vi "TCS_CFN_VS50BR_v2.vi"() -> ()   [LabVIEW 2011]
uses:
  <vilib>/Instr/_visa.llb/VISA Configure Serial Port (Instr).vi
panel:
  in  "LP_X-Up 4":sgl(slide) scale=-180.0..180.0
  in  "LP_Y-Easth 4":sgl(slide)=0.128098 scale=-180.0..180.0
  in  "LP_Z-North 4":sgl(slide)=0.467339 scale=-180.0..180.0
  in  "Height 4":sgl(slide)=622.367 scale=-2000.0..10000.0
  in  "Longitude 4":sgl(slide)=-45.860622 scale=-180.0..180.0
  in  "Latitude  2":sgl(slide)=-23.213156 scale=-90.0..90.0
  in  "Azimuth 4":sgl(slide) scale=0.0..360.0
  in  "Offset Pitch 4":sgl(slide) scale=-180.0..180.0
  in  "Offset Roll 4":sgl(slide) scale=-180.0..180.0
  in  "Offset Yaw 4":sgl(slide) scale=-180.0..180.0
  in  "Send":bool
  in  "LP_X-Up 3":sgl(slide) scale=-180.0..180.0
  in  "LP_Y-Easth 3":sgl(slide)=0.128098 scale=-180.0..180.0
  in  "LP_Z-North 3":sgl(slide)=0.467339 scale=-180.0..180.0
  in  "Height 3":sgl(slide)=622.367 scale=-2000.0..10000.0
  in  "Longitude 3":sgl(slide)=-45.860622 scale=-180.0..180.0
  in  "Latitude  2":sgl(slide)=-23.213156 scale=-90.0..90.0
  in  "Azimuth 3":sgl(slide) scale=0.0..360.0
  in  "Offset Pitch 3":sgl(slide) scale=-180.0..180.0
  in  "Offset Roll 3":sgl(slide) scale=-180.0..180.0
  in  "Offset Yaw 3":sgl(slide) scale=-180.0..180.0
  in  "Init":bool
  in  "LP_X-Up 2":sgl(slide) scale=-180.0..180.0
  in  "LP_Y-Easth 2":sgl(slide)=0.128098 scale=-180.0..180.0
  in  "LP_Z-North 2":sgl(slide)=0.467339 scale=-180.0..180.0
  in  "Height 2":sgl(slide)=622.367 scale=-2000.0..10000.0
  in  "Longitude 2":sgl(slide)=-45.860622 scale=-180.0..180.0
  in  "Latitude  2":sgl(slide)=-23.213156 scale=-90.0..90.0
  in  "Azimuth 2":sgl(slide) scale=0.0..360.0
  in  "Offset Pitch 2":sgl(slide) scale=-180.0..180.0
  in  "Offset Roll 2":sgl(slide) scale=-180.0..180.0
  in  "Offset Yaw 2":sgl(slide) scale=-180.0..180.0
  in  "Tab Control 4":enum32{"TCS_Utility", "TCS_Utility 2"}(tab)
  in  "Fact Reserved":bool
  in  "Download":bool
  in  "Fact Config":bool
  in  "NavOn":bool
  out "Half Second":bool[][](array[boolean])=[[FALSE, FALSE, FALSE, FALSE, FALSE, FALSE, FALSE, FALSE, FALSE, FALSE], [FALSE, FALSE, TRUE, TRUE, TRUE, TRUE, TRUE, FALSE, FALSE, FALSE], [FALSE, TRUE, FALSE, FALSE, FALSE, FALSE, FALSE, TRUE, FALSE, FALSE], [FALSE, TRUE, FALSE, FALSE, FALSE, FALSE, FALSE, TRUE, FALSE, FALSE], [FALSE, TRUE, FALSE, FALSE, FALSE, FALSE, FALSE, TRUE, FALSE, FALSE], [FALSE, TRUE, FALSE, FALSE, FALSE, FALSE, FALSE, TRUE, FALSE, FALSE], [FALSE, TRUE, FALSE, FALSE, FALSE, FALSE, FALSE, TRUE, FALSE, FALSE], [FALSE, TRUE, FALSE, FALSE, FALSE, FALSE, FALSE, TRUE, FALSE, FALSE], [FALSE, FALSE, TRUE, TRUE, TRUE, TRUE, TRUE, FALSE, FALSE, FALSE], [FALSE, FALSE, FALSE, FALSE, FALSE, FALSE, FALSE, FALSE, FALSE, FALSE]]
  out "Min 1":bool[][](array[boolean])=[[FALSE, FALSE, FALSE, FALSE, FALSE, FALSE, FALSE, FALSE, FALSE, FALSE], [FALSE, FALSE, TRUE, TRUE, TRUE, TRUE, TRUE, FALSE, FALSE, FALSE], [FALSE, TRUE, FALSE, FALSE, FALSE, FALSE, FALSE, TRUE, FALSE, FALSE], [FALSE, TRUE, FALSE, FALSE, FALSE, FALSE, FALSE, TRUE, FALSE, FALSE], [FALSE, TRUE, FALSE, FALSE, FALSE, FALSE, FALSE, TRUE, FALSE, FALSE], [FALSE, TRUE, FALSE, FALSE, FALSE, FALSE, FALSE, TRUE, FALSE, FALSE], [FALSE, TRUE, FALSE, FALSE, FALSE, FALSE, FALSE, TRUE, FALSE, FALSE], [FALSE, TRUE, FALSE, FALSE, FALSE, FALSE, FALSE, TRUE, FALSE, FALSE], [FALSE, FALSE, TRUE, TRUE, TRUE, TRUE, TRUE, FALSE, FALSE, FALSE], [FALSE, FALSE, FALSE, FALSE, FALSE, FALSE, FALSE, FALSE, FALSE, FALSE]]
  out "Min 0":bool[][](array[boolean])=[[FALSE, FALSE, FALSE, FALSE, FALSE, FALSE, FALSE, FALSE, FALSE, FALSE], [FALSE, FALSE, TRUE, TRUE, TRUE, TRUE, TRUE, FALSE, FALSE, FALSE], [FALSE, TRUE, FALSE, FALSE, FALSE, FALSE, FALSE, TRUE, FALSE, FALSE], [FALSE, TRUE, FALSE, FALSE, FALSE, FALSE, FALSE, TRUE, FALSE, FALSE], [FALSE, TRUE, FALSE, FALSE, FALSE, FALSE, FALSE, TRUE, FALSE, FALSE], [FALSE, TRUE, FALSE, FALSE, FALSE, FALSE, FALSE, TRUE, FALSE, FALSE], [FALSE, TRUE, FALSE, FALSE, FALSE, FALSE, FALSE, TRUE, FALSE, FALSE], [FALSE, TRUE, FALSE, FALSE, FALSE, FALSE, FALSE, TRUE, FALSE, FALSE], [FALSE, FALSE, TRUE, TRUE, TRUE, TRUE, TRUE, FALSE, FALSE, FALSE], [FALSE, FALSE, FALSE, FALSE, FALSE, FALSE, FALSE, FALSE, FALSE, FALSE]]
  out "Hour 1":bool[][](array[boolean])=[[FALSE, FALSE, FALSE, FALSE, FALSE, FALSE, FALSE, FALSE, FALSE, FALSE], [FALSE, FALSE, TRUE, TRUE, TRUE, TRUE, TRUE, FALSE, FALSE, FALSE], [FALSE, TRUE, FALSE, FALSE, FALSE, FALSE, FALSE, TRUE, FALSE, FALSE], [FALSE, TRUE, FALSE, FALSE, FALSE, FALSE, FALSE, TRUE, FALSE, FALSE], [FALSE, TRUE, FALSE, FALSE, FALSE, FALSE, FALSE, TRUE, FALSE, FALSE], [FALSE, TRUE, FALSE, FALSE, FALSE, FALSE, FALSE, TRUE, FALSE, FALSE], [FALSE, TRUE, FALSE, FALSE, FALSE, FALSE, FALSE, TRUE, FALSE, FALSE], [FALSE, TRUE, FALSE, FALSE, FALSE, FALSE, FALSE, TRUE, FALSE, FALSE], [FALSE, FALSE, TRUE, TRUE, TRUE, TRUE, TRUE, FALSE, FALSE, FALSE], [FALSE, FALSE, FALSE, FALSE, FALSE, FALSE, FALSE, FALSE, FALSE, FALSE]]
  out "Hour 0":bool[][](array[boolean])=[[FALSE, FALSE, FALSE, FALSE, FALSE, FALSE, FALSE, FALSE, FALSE, FALSE], [FALSE, FALSE, TRUE, TRUE, TRUE, TRUE, TRUE, FALSE, FALSE, FALSE], [FALSE, TRUE, FALSE, FALSE, FALSE, FALSE, FALSE, TRUE, FALSE, FALSE], [FALSE, TRUE, FALSE, FALSE, FALSE, FALSE, FALSE, TRUE, FALSE, FALSE], [FALSE, TRUE, FALSE, FALSE, FALSE, FALSE, FALSE, TRUE, FALSE, FALSE], [FALSE, TRUE, FALSE, FALSE, FALSE, FALSE, FALSE, TRUE, FALSE, FALSE], [FALSE, TRUE, FALSE, FALSE, FALSE, FALSE, FALSE, TRUE, FALSE, FALSE], [FALSE, TRUE, FALSE, FALSE, FALSE, FALSE, FALSE, TRUE, FALSE, FALSE], [FALSE, FALSE, TRUE, TRUE, TRUE, TRUE, TRUE, FALSE, FALSE, FALSE], [FALSE, FALSE, FALSE, FALSE, FALSE, FALSE, FALSE, FALSE, FALSE, FALSE]]
  in  "Stop":bool
  out "string in":string
  out "string out":string
  out "DV_Word":bool[](array[boolean])
  out "B_55":u8 format="%x"
  out "B_54":u8 format="%x"
  out "String":string
  in  "Tab Control":enum32{"Page 1", "Page 2", "Page 3"}(tab)
  in  "Offset Yaw":sgl(slide) scale=-180.0..180.0
  in  "Offset Roll":sgl(slide) scale=-180.0..180.0
  in  "Offset Pitch":sgl(slide) scale=-180.0..180.0
  in  "Longitude":sgl(slide)=-45.860622 scale=-180.0..180.0
  in  "Latitude":sgl(slide)=-23.213156 scale=-90.0..90.0
  in  "Azimuth":sgl(slide) scale=0.0..360.0
  in  "Height":sgl(slide)=622.367 scale=-2000.0..10000.0
  in  "LP_X-Up":sgl(slide) scale=-180.0..180.0
  in  "LP_Y-Easth":sgl(slide)=0.128098 scale=-180.0..180.0
  in  "LP_Z-North":sgl(slide)=0.467339 scale=-180.0..180.0
  # "B#55 (Configuration and Command Mode)"
  # "0x35"
  # "0xBD"
  # "0XFA"
  # "0XEE"
  # "0XAB"
  # "B#54 (Data Validity Word)"
  # "1= Installation Offset input valid data\n1= Launch Azimuth geodetic orientation, position, (lat, long, height) valid \n1= Velocity input valid data \nRFU\nRFU\nRFU\n 7,6     00= \"Init Cmd\" (Configuration parameters setting)\n           10= \"NAV_On\"\n           01= Reserved\n           11= Enter Configuration Mode"
  # "0\n1\n2\n3\n4\n5\n6\n7"
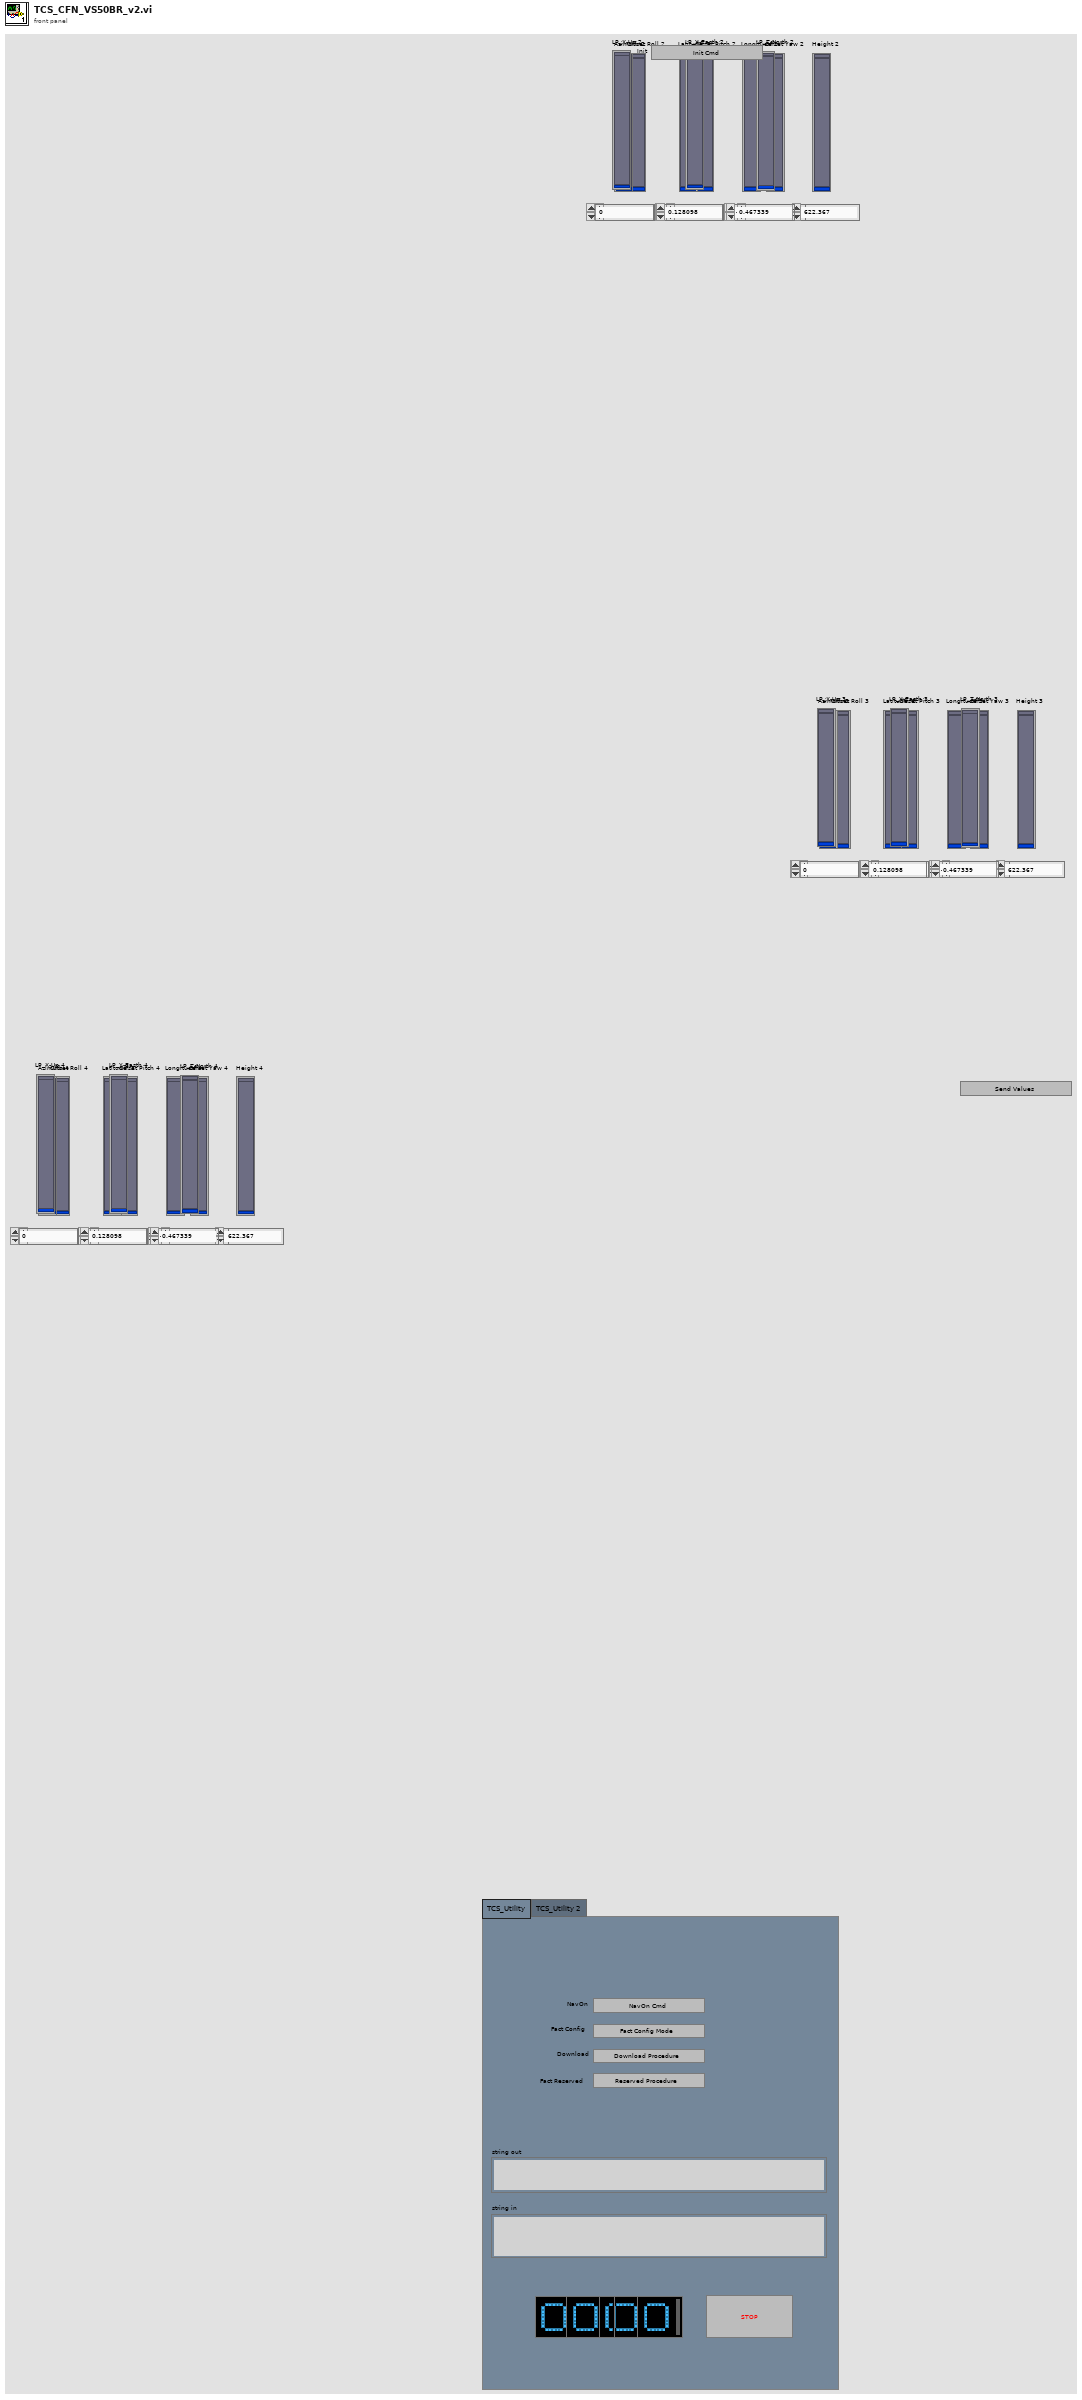
[diagram p1: front panel]
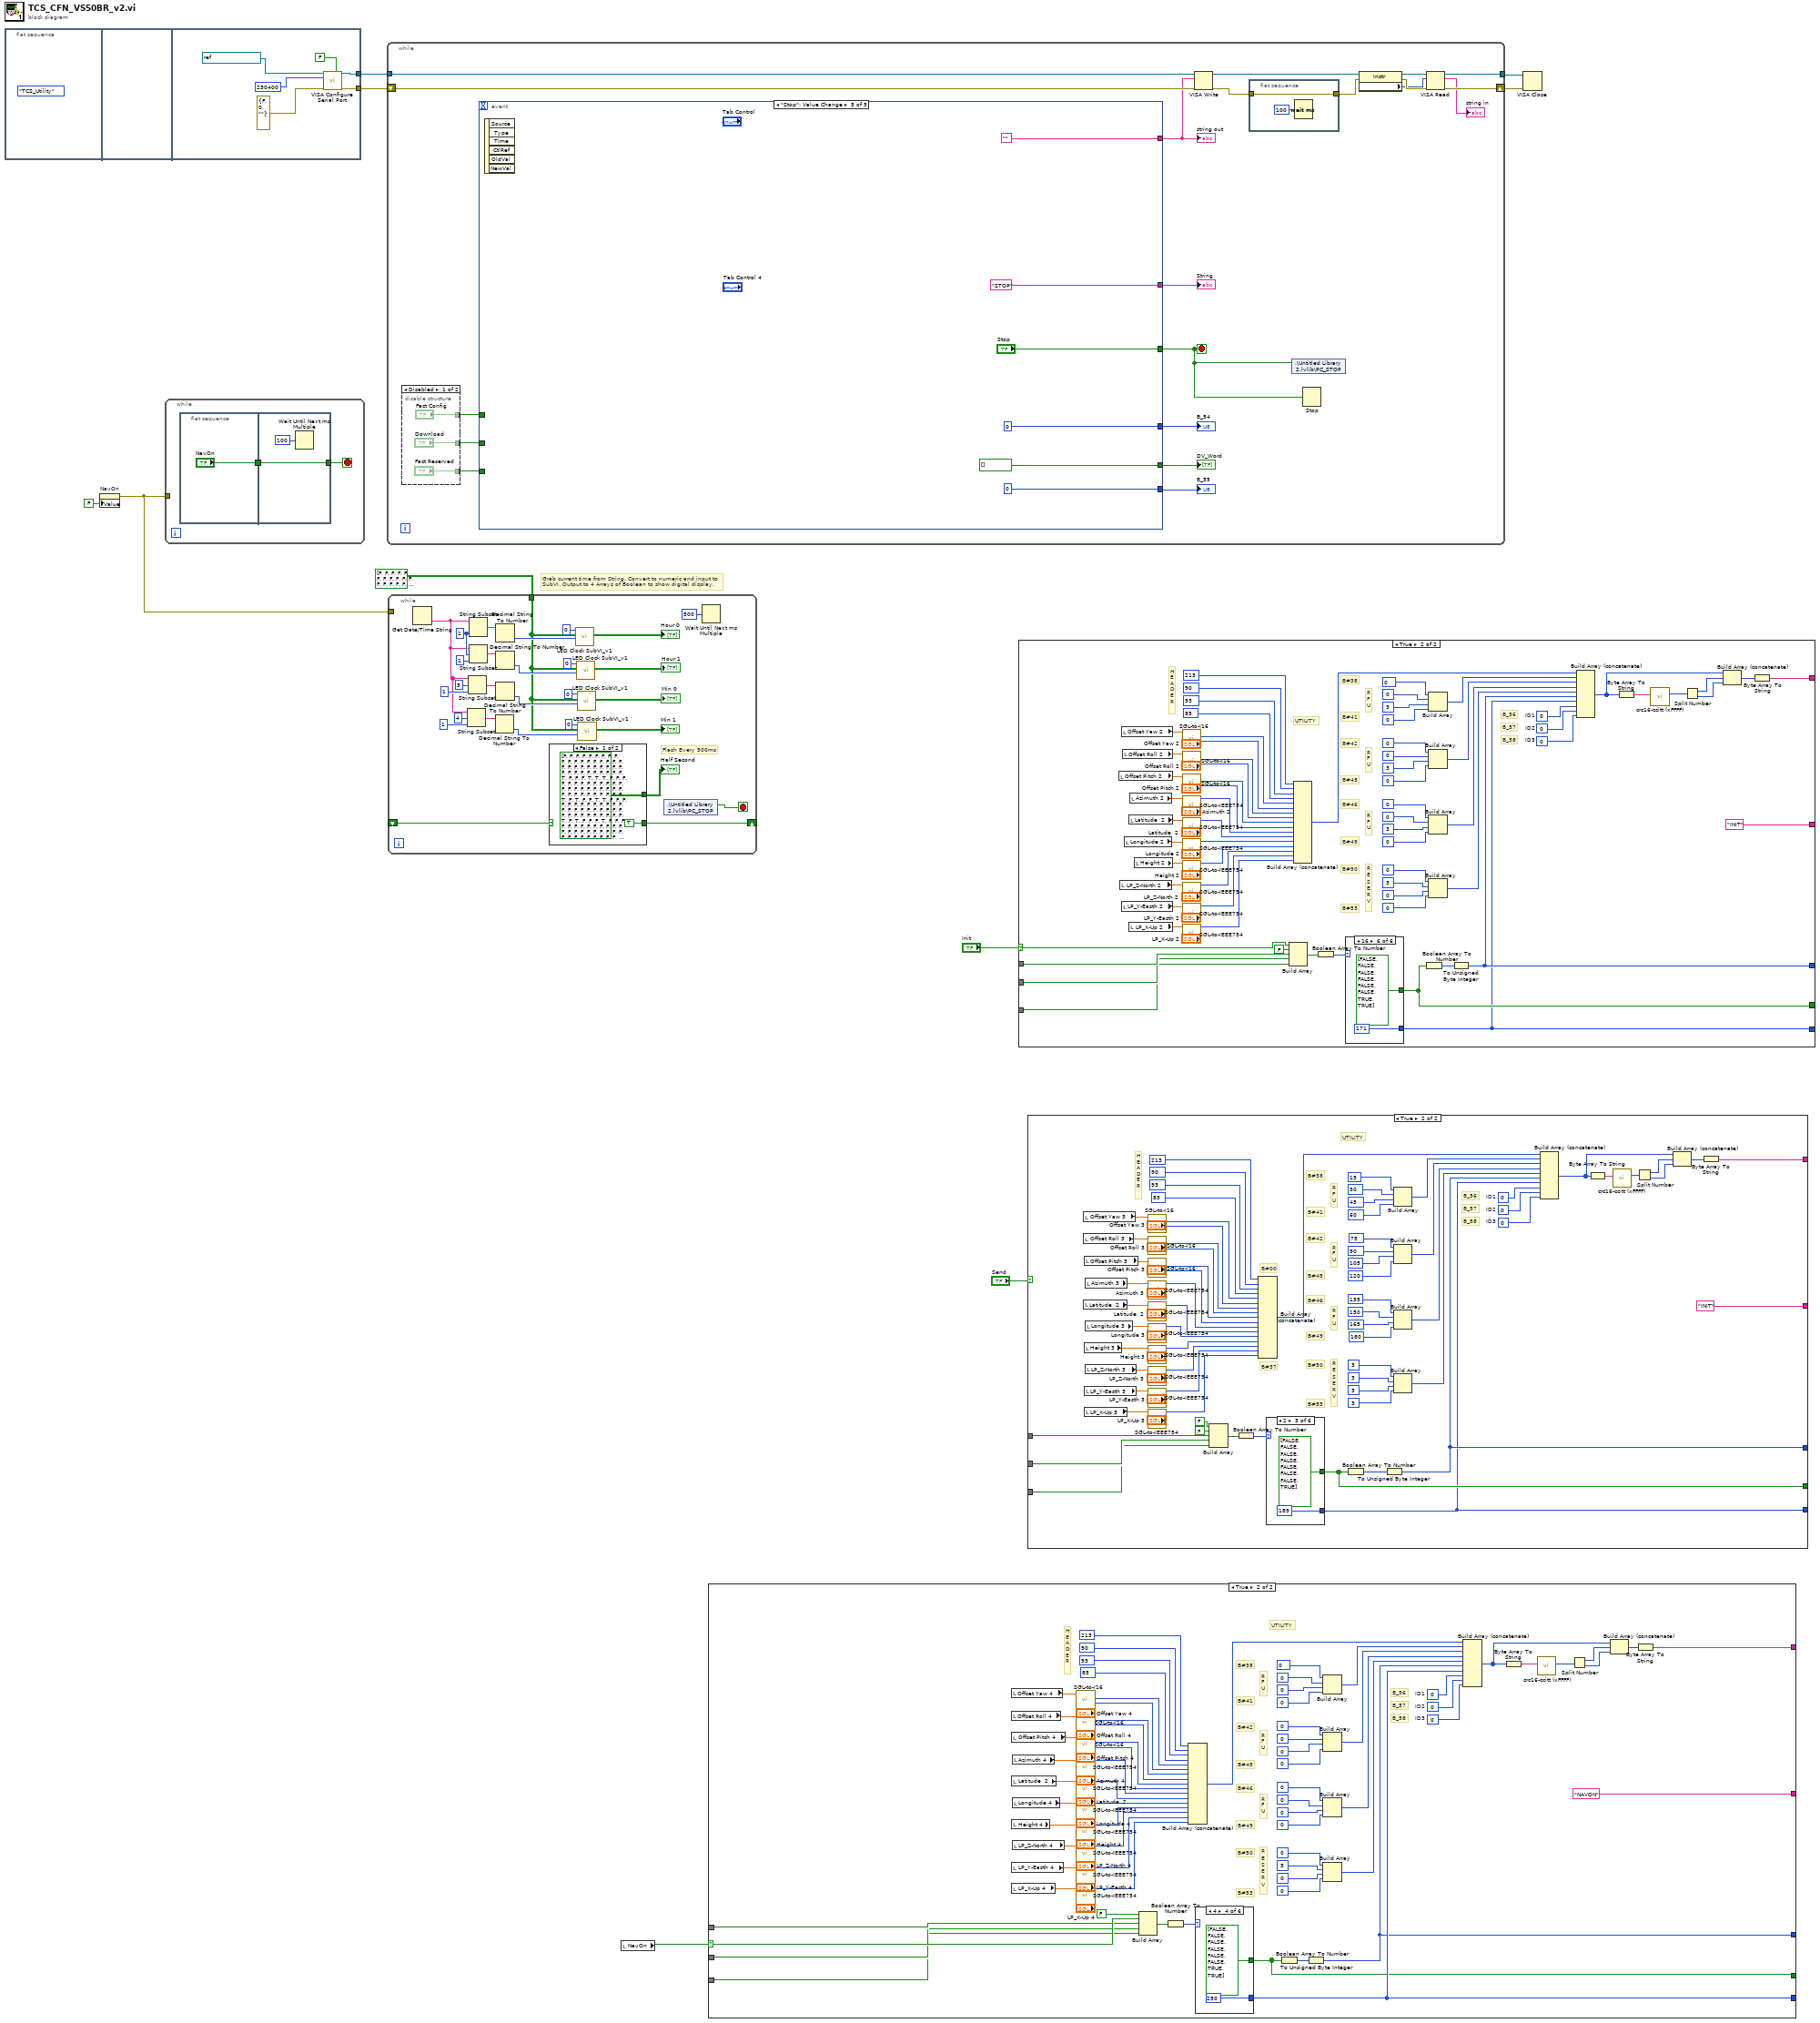
[diagram p0: block diagram]
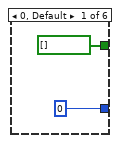
[diagram p3: hidden frame]
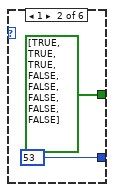
[diagram p4: hidden frame]
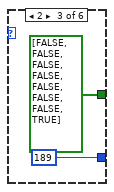
[diagram p5: hidden frame]
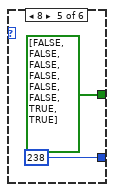
[diagram p6: hidden frame]
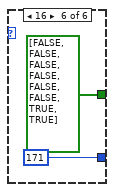
[diagram p7: hidden frame]
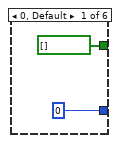
[diagram p9: hidden frame]
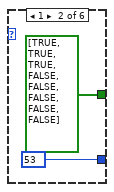
[diagram p10: hidden frame]
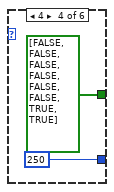
[diagram p11: hidden frame]
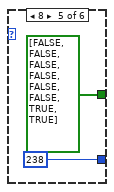
[diagram p12: hidden frame]
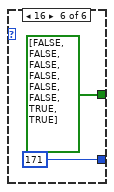
[diagram p13: hidden frame]
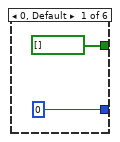
[diagram p15: hidden frame]
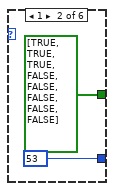
[diagram p16: hidden frame]
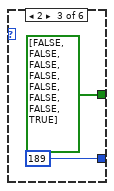
[diagram p17: hidden frame]
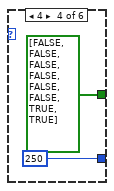
[diagram p18: hidden frame]
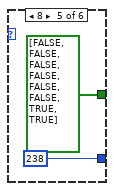
[diagram p19: hidden frame]
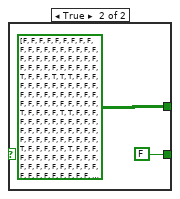
[diagram p20: hidden frame]
diagram:
  # "Grab current time from String, Convert to numeric and input to\nSubVI. Output to 4 Arrays of Boolean to show digital display."
  n1 = flat-sequence {
    tunnel: [w13] -> w10
    tunnel: [w12] -> w9
    frame #0 {
      (unwired) enum32{"TCS_Utility", "Parser"}."TCS_Utility" ("Tab Control 3")
    }
    frame #1 {
    }
    frame #2 {
      n2 = call-poly "VISA Configure Serial Port"("VISA resource name"=refnum<visa-resource-name> "ASRL3::INSTR", "Enable Termination\nChar (T)"=FALSE ("Enable Termination\nChar (T)"), "baud rate (9600)"=u32 230400 ("Serial Settings:Baud Rate"), "error in (no error)"=errorcluster {"status"=FALSE, "code"=0, "source"=""}) -> ("VISA resource name out"=w13:refnum<visa-resource-name>, "error out"=w12:errorcluster)  [unwired: 10 in]
    }
  }
  n3 = property on="NavOn" class="Bool (strict)"("Value"=FALSE ("NavOn")) -> (error out=w4:errorcluster)  [unwired: 2 in, 1 out]
  n4 = while {
    tunnel: w4 -> [_]
    stop <- w18 stop-if-true
    n5 = flat-sequence {
      tunnel: ["NavOn"] -> w17
      tunnel: [w20] -> w18
      tunnel: w17 -> [w20]
      frame #0 {
      }
      frame #1 {
        n6 = Wait Until Next ms Multiple(millisecond multiple=u32 100) -> ()  [unwired: 1 out]
      }
    }
  }
  n7 = while {
    tunnel: w10 -> [w34]
    tunnel: [w24] -> w8
    shift-right: [w25] -> w7
    shift-left: w9 -> [w33]
    stop <- w22 stop-if-true
    n8 = disable-structure shown="Disabled" {
      disable-tunnel: ["Fact Config" _] -> w41
      disable-tunnel: ["Download" _] -> w40
      disable-tunnel: ["Fact Reserved" _] -> w39
      frame Disabled {
      }
      frame Enabled {
      }
    }
    n9 = event shown="[4] \"Stop\": Value Change" {
      selector: _ -> [_ _ _ _ _]
      dyn-events: _ -> [_ _ _ _ _]
      timeout: _ -> [_ _ _ _ _]
      tunnel: ["" _ w50 w51 ""] -> w32
      tunnel: w41 -> [_ _ _ _ _]
      tunnel: w40 -> [_ _ _ _ _]
      tunnel: w39 -> [_ _ _ _ _]
      tunnel: [u8 0 _ _ _ u8 0] -> w38
      tunnel: [bool[] [] ("DV_Word") _ _ _ bool[] [] ("DV_Word")] -> w37
      tunnel: [u8 0 _ _ _ u8 0] -> w36
      tunnel: [_ _ _ _ "Stop"] -> w22
      tunnel: ["TIMEOUT" _ w49 _ "STOP"] -> w35
      event Timeout {
        n10 = event-data() -> ()  [unwired: 1 in, 3 out]
      }
      event #1 (no event record) {
        n11 = event-data() -> ()  [unwired: 1 in, 6 out]
      }
      event #2 (no event record) {
        n12 = event-data() -> ()  [unwired: 1 in, 6 out]
      }
      event "NavOn": Value Change {
        n13 = event-data() -> ()  [unwired: 1 in, 6 out]
      }
      event "Stop": Value Change {
        n14 = event-data() -> ()  [unwired: 1 in, 6 out]
      }
    }
    "string out" <- w32
    "B_54" <- w38
    "DV_Word" <- w37
    "B_55" <- w36
    "String" <- w35
    n15 = VISA Write(VISA resource name=w34, write buffer=w32, error in (no error)=w33) -> (VISA resource name out=w31:refnum<visa-resource-name>, error out=w29:errorcluster)  [unwired: 1 out]
    n16 = flat-sequence {
      tunnel: [w42] -> w30
      tunnel: w29 -> [w42]
      frame #0 {
        n17 = Wait (ms)(milliseconds to wait=u32 100) -> ()  [unwired: 1 out]
      }
    }
    n18 = shared-variable ".\\Untitled Library 2.lvlib\\PC_STOP"(w22) -> ()  [unwired: 1 in, 1 out]
    n19 = Stop(stop? (T)=w22) -> ()
    n20 = property class="Instr"(reference=w31, error in=w30) -> (reference out=w28:refnum<visa-resource-name>, error out=w27:errorcluster, "Serial Settings:Number of Bytes at Serial Port"=w26:u32)
    n21 = VISA Read(VISA resource name=w28, byte count=w26, error in (no error)=w27) -> (VISA resource name out=w24:refnum<visa-resource-name>, read buffer=→"string in":string, error out=w25:errorcluster)  [unwired: 1 out]
  }
  n22 = while {
    tunnel: bool[][] [[FALSE, FALSE, FALSE, FALSE, FALSE, FALSE, FALSE, FALSE, FALSE, FALSE, FALSE, FALSE, FALSE, FALSE, FALSE, FALSE, FALSE, FALSE, FALSE, FALSE, FALSE, FALSE, FALSE, FALSE, FALSE, FALSE, FALSE, FALSE, FALSE, FALSE, FALSE, FALSE, FALSE, FALSE, FALSE, FALSE, FALSE, FALSE, FALSE, TRUE], [FALSE, FALSE, FALSE, TRUE, TRUE, TRUE, FALSE, FALSE, FALSE, FALSE, FALSE, FALSE, FALSE, FALSE, FALSE, FALSE, FALSE, FALSE, FALSE, FALSE, FALSE, FALSE, FALSE, FALSE, FALSE, FALSE, FALSE, FALSE, FALSE, FALSE, FALSE, FALSE, FALSE, FALSE, FALSE, FALSE, FALSE, FALSE, FALSE, TRUE], [FALSE, FALSE, FALSE, FALSE, TRUE, TRUE, FALSE, FALSE, FALSE, FALSE, FALSE, FALSE, FALSE, FALSE, FALSE, FALSE, FALSE, FALSE, FALSE, FALSE, FALSE, FALSE, FALSE, FALSE, FALSE, FALSE, FALSE, FALSE, FALSE, FALSE, FALSE, FALSE, FALSE, FALSE, FALSE, FALSE, FALSE, FALSE, FALSE, TRUE], [FALSE, FALSE, FALSE, FALSE, FALSE, TRUE, FALSE, FALSE, FALSE, FALSE, FALSE, FALSE, FALSE, FALSE, FALSE, FALSE, FALSE, FALSE, FALSE, FALSE, FALSE, FALSE, FALSE, FALSE, FALSE, FALSE, FALSE, FALSE, FALSE, FALSE, FALSE, FALSE, FALSE, FALSE, FALSE, FALSE, FALSE, FALSE, FALSE, TRUE], [FALSE, FALSE, FALSE, FALSE, FALSE, TRUE, FALSE, FALSE, FALSE, FALSE, FALSE, FALSE, FALSE, FALSE, FALSE, FALSE, FALSE, FALSE, FALSE, FALSE, FALSE, FALSE, FALSE, FALSE, FALSE, FALSE, FALSE, FALSE, FALSE, FALSE, FALSE, FALSE, FALSE, FALSE, FALSE, FALSE, FALSE, FALSE, FALSE, TRUE], [FALSE, FALSE, FALSE, FALSE, FALSE, TRUE, FALSE, FALSE, FALSE, FALSE, FALSE, FALSE, FALSE, FALSE, FALSE, FALSE, FALSE, FALSE, FALSE, FALSE, FALSE, FALSE, FALSE, FALSE, FALSE, FALSE, FALSE, FALSE, FALSE, FALSE, FALSE, FALSE, FALSE, FALSE, FALSE, FALSE, FALSE, FALSE, FALSE, TRUE], [FALSE, FALSE, FALSE, FALSE, FALSE, TRUE, FALSE, FALSE, FALSE, FALSE, FALSE, FALSE, FALSE, FALSE, FALSE, FALSE, FALSE, FALSE, FALSE, FALSE, FALSE, FALSE, FALSE, FALSE, FALSE, FALSE, FALSE, FALSE, FALSE, FALSE, FALSE, FALSE, FALSE, FALSE, FALSE, FALSE, FALSE, FALSE, FALSE, TRUE], [FALSE, FALSE, FALSE, FALSE, FALSE, TRUE, FALSE, FALSE, FALSE, FALSE, FALSE, FALSE, FALSE, FALSE, FALSE, FALSE, FALSE, FALSE, FALSE, FALSE, FALSE, FALSE, FALSE, FALSE, FALSE, FALSE, FALSE, FALSE, FALSE, FALSE, FALSE, FALSE, FALSE, FALSE, FALSE, FALSE, FALSE, FALSE, FALSE, TRUE], [FALSE, FALSE, FALSE, TRUE, TRUE, TRUE, TRUE, TRUE, FALSE, FALSE, FALSE, FALSE, FALSE, FALSE, FALSE, FALSE, FALSE, FALSE, FALSE, FALSE, FALSE, FALSE, FALSE, FALSE, FALSE, FALSE, FALSE, FALSE, FALSE, FALSE, FALSE, FALSE, FALSE, FALSE, FALSE, FALSE, FALSE, FALSE, FALSE, TRUE], [FALSE, FALSE, FALSE, FALSE, FALSE, FALSE, FALSE, FALSE, FALSE, FALSE, FALSE, FALSE, FALSE, FALSE, FALSE, FALSE, FALSE, FALSE, FALSE, FALSE, FALSE, FALSE, FALSE, FALSE, FALSE, FALSE, FALSE, FALSE, FALSE, FALSE, FALSE, FALSE, FALSE, FALSE, FALSE, FALSE, FALSE, FALSE, FALSE, TRUE]] ("Base Array") -> [w66]
    shift-right: [w62] -> _
    shift-left: _ -> [w63]
    tunnel: w4 -> [_]
    stop <- w61 stop-if-true
    w79 = 1 ("length (rest)")
    # "Flash Every 500ms"
    n23 = Get Date/Time String() -> (time string=w71:string)  [unwired: 3 in, 1 out]
    n24 = String Subset(string=w71, offset (0)=4, length (rest)=1 ("length (rest)")) -> (substring=w68:string)
    n25 = String Subset(string=w71, offset (0)=3, length (rest)=1 ("length (rest)")) -> (substring=w74:string)
    n26 = String Subset(string=w71, length (rest)=w79) -> (substring=w81:string)  [unwired: 1 in]
    n27 = String Subset(string=w71, offset (0)=w79, length (rest)=1 ("length (rest)")) -> (substring=w76:string)
    n28 = Decimal String To Number(string=w68) -> (number=w67:i32)  [unwired: 2 in, 1 out]
    n29 = Decimal String To Number(string=w81) -> (number=w80:i32)  [unwired: 2 in, 1 out]
    n30 = Decimal String To Number(string=w76) -> (number=w75:i32)  [unwired: 2 in, 1 out]
    n31 = Decimal String To Number(string=w74) -> (number=w73:i32)  [unwired: 2 in, 1 out]
    n32 = case shown="False" w63 {
      tunnel: [bool[][] [[FALSE, FALSE, FALSE, FALSE, FALSE, FALSE, FALSE, FALSE, FALSE, FALSE, FALSE, FALSE, FALSE, FALSE, FALSE, FALSE, FALSE, FALSE, FALSE, FALSE, FALSE, FALSE, FALSE, FALSE, FALSE, FALSE, FALSE, FALSE, FALSE, FALSE, FALSE, FALSE, FALSE, FALSE, FALSE, FALSE, FALSE, FALSE, FALSE, TRUE], [FALSE, FALSE, FALSE, TRUE, TRUE, TRUE, FALSE, FALSE, FALSE, FALSE, FALSE, FALSE, FALSE, FALSE, FALSE, FALSE, FALSE, FALSE, FALSE, FALSE, FALSE, FALSE, FALSE, FALSE, FALSE, FALSE, FALSE, FALSE, FALSE, FALSE, FALSE, FALSE, FALSE, FALSE, FALSE, FALSE, FALSE, FALSE, FALSE, TRUE], [FALSE, TRUE, FALSE, FALSE, TRUE, TRUE, FALSE, FALSE, FALSE, FALSE, FALSE, FALSE, FALSE, FALSE, FALSE, FALSE, FALSE, FALSE, FALSE, FALSE, FALSE, FALSE, FALSE, FALSE, FALSE, FALSE, FALSE, FALSE, FALSE, FALSE, FALSE, FALSE, FALSE, FALSE, FALSE, FALSE, FALSE, FALSE, FALSE, TRUE], [FALSE, TRUE, FALSE, FALSE, FALSE, TRUE, FALSE, FALSE, FALSE, FALSE, FALSE, FALSE, FALSE, FALSE, FALSE, FALSE, FALSE, FALSE, FALSE, FALSE, FALSE, FALSE, FALSE, FALSE, FALSE, FALSE, FALSE, FALSE, FALSE, FALSE, FALSE, FALSE, FALSE, FALSE, FALSE, FALSE, FALSE, FALSE, FALSE, TRUE], [FALSE, FALSE, FALSE, FALSE, FALSE, TRUE, FALSE, FALSE, FALSE, FALSE, FALSE, FALSE, FALSE, FALSE, FALSE, FALSE, FALSE, FALSE, FALSE, FALSE, FALSE, FALSE, FALSE, FALSE, FALSE, FALSE, FALSE, FALSE, FALSE, FALSE, FALSE, FALSE, FALSE, FALSE, FALSE, FALSE, FALSE, FALSE, FALSE, TRUE], [FALSE, FALSE, FALSE, FALSE, FALSE, TRUE, FALSE, FALSE, FALSE, FALSE, FALSE, FALSE, FALSE, FALSE, FALSE, FALSE, FALSE, FALSE, FALSE, FALSE, FALSE, FALSE, FALSE, FALSE, FALSE, FALSE, FALSE, FALSE, FALSE, FALSE, FALSE, FALSE, FALSE, FALSE, FALSE, FALSE, FALSE, FALSE, FALSE, TRUE], [FALSE, TRUE, FALSE, FALSE, FALSE, TRUE, FALSE, FALSE, FALSE, FALSE, FALSE, FALSE, FALSE, FALSE, FALSE, FALSE, FALSE, FALSE, FALSE, FALSE, FALSE, FALSE, FALSE, FALSE, FALSE, FALSE, FALSE, FALSE, FALSE, FALSE, FALSE, FALSE, FALSE, FALSE, FALSE, FALSE, FALSE, FALSE, FALSE, TRUE], [FALSE, TRUE, FALSE, FALSE, FALSE, TRUE, FALSE, FALSE, FALSE, FALSE, FALSE, FALSE, FALSE, FALSE, FALSE, FALSE, FALSE, FALSE, FALSE, FALSE, FALSE, FALSE, FALSE, FALSE, FALSE, FALSE, FALSE, FALSE, FALSE, FALSE, FALSE, FALSE, FALSE, FALSE, FALSE, FALSE, FALSE, FALSE, FALSE, TRUE], [FALSE, FALSE, FALSE, TRUE, TRUE, TRUE, TRUE, TRUE, FALSE, FALSE, FALSE, FALSE, FALSE, FALSE, FALSE, FALSE, FALSE, FALSE, FALSE, FALSE, FALSE, FALSE, FALSE, FALSE, FALSE, FALSE, FALSE, FALSE, FALSE, FALSE, FALSE, FALSE, FALSE, FALSE, FALSE, FALSE, FALSE, FALSE, FALSE, TRUE], [FALSE, FALSE, FALSE, FALSE, FALSE, FALSE, FALSE, FALSE, FALSE, FALSE, FALSE, FALSE, FALSE, FALSE, FALSE, FALSE, FALSE, FALSE, FALSE, FALSE, FALSE, FALSE, FALSE, FALSE, FALSE, FALSE, FALSE, FALSE, FALSE, FALSE, FALSE, FALSE, FALSE, FALSE, FALSE, FALSE, FALSE, FALSE, FALSE, TRUE]] ("Base Array 2") bool[][] [[FALSE, FALSE, FALSE, FALSE, FALSE, FALSE, FALSE, FALSE, FALSE, FALSE, FALSE, FALSE, FALSE, FALSE, FALSE, FALSE, FALSE, FALSE, FALSE, FALSE, FALSE, FALSE, FALSE, FALSE, FALSE, FALSE, FALSE, FALSE, FALSE, FALSE, FALSE, FALSE, FALSE, FALSE, FALSE, FALSE, FALSE, FALSE, FALSE, TRUE], [FALSE, FALSE, FALSE, TRUE, TRUE, TRUE, FALSE, FALSE, FALSE, FALSE, FALSE, FALSE, FALSE, FALSE, FALSE, FALSE, FALSE, FALSE, FALSE, FALSE, FALSE, FALSE, FALSE, FALSE, FALSE, FALSE, FALSE, FALSE, FALSE, FALSE, FALSE, FALSE, FALSE, FALSE, FALSE, FALSE, FALSE, FALSE, FALSE, TRUE], [FALSE, FALSE, FALSE, FALSE, TRUE, TRUE, FALSE, FALSE, FALSE, FALSE, FALSE, FALSE, FALSE, FALSE, FALSE, FALSE, FALSE, FALSE, FALSE, FALSE, FALSE, FALSE, FALSE, FALSE, FALSE, FALSE, FALSE, FALSE, FALSE, FALSE, FALSE, FALSE, FALSE, FALSE, FALSE, FALSE, FALSE, FALSE, FALSE, TRUE], [FALSE, FALSE, FALSE, FALSE, FALSE, TRUE, FALSE, FALSE, FALSE, FALSE, FALSE, FALSE, FALSE, FALSE, FALSE, FALSE, FALSE, FALSE, FALSE, FALSE, FALSE, FALSE, FALSE, FALSE, FALSE, FALSE, FALSE, FALSE, FALSE, FALSE, FALSE, FALSE, FALSE, FALSE, FALSE, FALSE, FALSE, FALSE, FALSE, TRUE], [FALSE, FALSE, FALSE, FALSE, FALSE, TRUE, FALSE, FALSE, FALSE, FALSE, FALSE, FALSE, FALSE, FALSE, FALSE, FALSE, FALSE, FALSE, FALSE, FALSE, FALSE, FALSE, FALSE, FALSE, FALSE, FALSE, FALSE, FALSE, FALSE, FALSE, FALSE, FALSE, FALSE, FALSE, FALSE, FALSE, FALSE, FALSE, FALSE, TRUE], [FALSE, FALSE, FALSE, FALSE, FALSE, TRUE, FALSE, FALSE, FALSE, FALSE, FALSE, FALSE, FALSE, FALSE, FALSE, FALSE, FALSE, FALSE, FALSE, FALSE, FALSE, FALSE, FALSE, FALSE, FALSE, FALSE, FALSE, FALSE, FALSE, FALSE, FALSE, FALSE, FALSE, FALSE, FALSE, FALSE, FALSE, FALSE, FALSE, TRUE], [FALSE, FALSE, FALSE, FALSE, FALSE, TRUE, FALSE, FALSE, FALSE, FALSE, FALSE, FALSE, FALSE, FALSE, FALSE, FALSE, FALSE, FALSE, FALSE, FALSE, FALSE, FALSE, FALSE, FALSE, FALSE, FALSE, FALSE, FALSE, FALSE, FALSE, FALSE, FALSE, FALSE, FALSE, FALSE, FALSE, FALSE, FALSE, FALSE, TRUE], [FALSE, FALSE, FALSE, FALSE, FALSE, TRUE, FALSE, FALSE, FALSE, FALSE, FALSE, FALSE, FALSE, FALSE, FALSE, FALSE, FALSE, FALSE, FALSE, FALSE, FALSE, FALSE, FALSE, FALSE, FALSE, FALSE, FALSE, FALSE, FALSE, FALSE, FALSE, FALSE, FALSE, FALSE, FALSE, FALSE, FALSE, FALSE, FALSE, TRUE], [FALSE, FALSE, FALSE, TRUE, TRUE, TRUE, TRUE, TRUE, FALSE, FALSE, FALSE, FALSE, FALSE, FALSE, FALSE, FALSE, FALSE, FALSE, FALSE, FALSE, FALSE, FALSE, FALSE, FALSE, FALSE, FALSE, FALSE, FALSE, FALSE, FALSE, FALSE, FALSE, FALSE, FALSE, FALSE, FALSE, FALSE, FALSE, FALSE, TRUE], [FALSE, FALSE, FALSE, FALSE, FALSE, FALSE, FALSE, FALSE, FALSE, FALSE, FALSE, FALSE, FALSE, FALSE, FALSE, FALSE, FALSE, FALSE, FALSE, FALSE, FALSE, FALSE, FALSE, FALSE, FALSE, FALSE, FALSE, FALSE, FALSE, FALSE, FALSE, FALSE, FALSE, FALSE, FALSE, FALSE, FALSE, FALSE, FALSE, TRUE]] ("Base Array 2")] -> w64
      tunnel: [TRUE FALSE] -> w62
      frame False {
      }
      frame True {
      }
    }
    "Half Second" <- w64
    n33 = call "LED Clock SubVI_v1.vi"("Number"=w80, "Array"=w66, "Position"=0) -> ("Time Out"=→"Hour 0":bool[][])  [unwired: 8 in]
    n34 = call "LED Clock SubVI_v1.vi"("Number"=w75, "Array"=w66, "Position"=0) -> ("Time Out"=→"Hour 1":bool[][])  [unwired: 8 in]
    n35 = call "LED Clock SubVI_v1.vi"("Number"=w73, "Array"=w66, "Position"=0) -> ("Time Out"=→"Min 0":bool[][])  [unwired: 8 in]
    n36 = call "LED Clock SubVI_v1.vi"("Number"=w67, "Array"=w66, "Position"=0) -> ("Time Out"=→"Min 1":bool[][])  [unwired: 8 in]
    n37 = shared-variable ".\\Untitled Library 2.lvlib\\PC_STOP"() -> (w61:bool)  [unwired: 1 in, 1 out]
    n38 = Wait Until Next ms Multiple(millisecond multiple=u32 500) -> ()  [unwired: 1 out]
  }
  n39 = local read "NavOn"() -> (w1:bool)
  n40 = case shown="True" w1 {
    selector: w1 -> [_ w102]
    tunnel: [_ w101] -> _
    tunnel: [_ w100] -> _
    tunnel: [_ w99] -> _
    tunnel: [_ w98] -> _
    tunnel: [_ w97] -> _
    tunnel: [_ w96] -> _
    tunnel: [_ "NAVON"] -> _
    tunnel: [_ w94] -> _
    frame False {
    }
    frame True {
      w120 = u8 0  # ID3
      w121 = u8 0  # ID2
      w122 = u8 0  # ID1
      # "B#53"
      # "B#50"
      # "B#49"
      # "B#46"
      # "B#45"
      # "B#42"
      # "B#41"
      # "B#38"
      # "B_58"
      # "B_57"
      # "B_56"
      # "R\nE\nS\nE\nR\nV"
      # "R\nF\nU"
      # "R\nF\nU"
      # "R\nF\nU"
      # "H\nE\nA\nD\nE\nR"
      # "UTILITY"
      n41 = local read "Offset Yaw 4"() -> (w112:sgl)
      n42 = local read "Offset Roll 4"() -> (w111:sgl)
      n43 = local read "Offset Pitch 4"() -> (w110:sgl)
      n44 = local read "Latitude  2"() -> (w108:sgl)
      n45 = local read "Height 4"() -> (w106:sgl)
      n46 = local read "LP_Y-Easth 4"() -> (w104:sgl)
      n47 = local read "LP_X-Up 4"() -> (w103:sgl)
      n48 = local read "Azimuth 4"() -> (w109:sgl)
      n49 = local read "Longitude 4"() -> (w107:sgl)
      n50 = local read "LP_Z-North 4"() -> (w105:sgl)
      n51 = call "SGL-to-I16.vi"("Range"=w112) -> ("lo(x)"=w155:u8, "hi(x)"=w156:u8)  [unwired: 8 in, 1 out]
      n52 = call "SGL-to-I16.vi"("Range"=w111) -> ("lo(x)"=w153:u8, "hi(x)"=w154:u8)  [unwired: 8 in, 1 out]
      n53 = call "SGL-to-I16.vi"("Range"=w110) -> ("lo(x)"=w151:u8, "hi(x)"=w152:u8)  [unwired: 8 in, 1 out]
      n54 = call "SGL-to-IEEE754.vi"("Input_DBL"=w109) -> ("Output_U8"=w150:u8[])  [unwired: 10 in]
      n55 = call "SGL-to-IEEE754.vi"("Input_DBL"=w108) -> ("Output_U8"=w149:u8[])  [unwired: 10 in]
      n56 = call "SGL-to-IEEE754.vi"("Input_DBL"=w107) -> ("Output_U8"=w148:u8[])  [unwired: 10 in]
      n57 = call "SGL-to-IEEE754.vi"("Input_DBL"=w106) -> ("Output_U8"=w147:u8[])  [unwired: 10 in]
      n58 = call "SGL-to-IEEE754.vi"("Input_DBL"=w105) -> ("Output_U8"=w146:u8[])  [unwired: 10 in]
      n59 = call "SGL-to-IEEE754.vi"("Input_DBL"=w104) -> ("Output_U8"=w145:u8[])  [unwired: 10 in]
      n60 = call "SGL-to-IEEE754.vi"("Input_DBL"=w103) -> ("Output_U8"=w144:u8[])  [unwired: 10 in]
      n61 = Build Array(FALSE ("element"), w102) -> (w162:bool[], w101:bool, w100:bool, w99:bool)
      n62 = Boolean Array To Number(Boolean array=w162) -> (number=w161:u32)
      n63 = Build Array (concatenate)(u8 213, u8 90, u8 93, u8 85, w156, w155, w154, w153, w152, w151, w150, w149, w148, w147, w146, w145, w144) -> (w127:u8[])
      n64 = case shown="4" w161 {
        tunnel: [u8 0 u8 53 u8 189 u8 250 u8 238 u8 171] -> w98
        tunnel: [bool[] [] ("DV_Word") bool[] [TRUE, TRUE, TRUE, FALSE, FALSE, FALSE, FALSE, FALSE] ("DV_Word") bool[] [FALSE, FALSE, FALSE, FALSE, FALSE, FALSE, FALSE, TRUE] ("DV_Word") bool[] [FALSE, FALSE, FALSE, FALSE, FALSE, FALSE, TRUE, TRUE] ("DV_Word") bool[] [FALSE, FALSE, FALSE, FALSE, FALSE, FALSE, TRUE, TRUE] ("DV_Word") bool[] [FALSE, FALSE, FALSE, FALSE, FALSE, FALSE, TRUE, TRUE] ("DV_Word")] -> w97
        frame 0, Default {
        }
        frame 1 {
        }
        frame 2 {
        }
        frame 4 {
        }
        frame 8 {
        }
        frame 16 {
        }
      }
      n65 = Boolean Array To Number(Boolean array=w97) -> (number=w163:u32)
      n66 = To Unsigned Byte Integer(number=w163) -> (unsigned 8bit integer=w96:u8)
      n67 = Build Array(u8 0, u8 0, u8 0, u8 0) -> (w126:u8[])
      n68 = Build Array(u8 0, u8 0, u8 0, u8 0) -> (w125:u8[])
      n69 = Build Array(u8 0, u8 0, u8 0, u8 0) -> (w124:u8[])
      n70 = Build Array(u8 0, u8 3, u8 0, u8 0) -> (w123:u8[])
      n71 = Build Array (concatenate)(w127, w126, w125, w124, w123, w96, w98, w122, w121, w120) -> (w117:u8[])
      n72 = Byte Array To String(unsigned byte array=w117) -> (string=w119:string)
      n73 = call "crc16-ccitt (xFFFF).vi"("Message"=w119) -> ("CRC"=w118:u16)  [unwired: 9 in, 1 out]
      n74 = Split Number(x=w118) -> (hi(x)=w116:u8, lo(x)=w115:u8)
      n75 = Build Array (concatenate)(w117, w116, w115) -> (w114:u8[])
      n76 = Byte Array To String(unsigned byte array=w114) -> (string=w94:string)
    }
  }
  n77 = case shown="True" "Init" {
    selector: "Init" -> [_ w179]
    tunnel: [_ w184] -> _
    tunnel: [_ "INIT"] -> _
    tunnel: [_ w182] -> _
    tunnel: [_ w181] -> _
    tunnel: [_ w180] -> _
    tunnel: [_ w178] -> _
    tunnel: [_ w177] -> _
    tunnel: [_ w176] -> _
    frame False {
    }
    frame True {
      w202 = u8 0  # ID3
      w203 = u8 0  # ID2
      w204 = u8 0  # ID1
      # "B#53"
      # "B#50"
      # "B#49"
      # "B#46"
      # "B#45"
      # "B#42"
      # "B#41"
      # "B#38"
      # "B_58"
      # "B_57"
      # "B_56"
      # "R\nE\nS\nE\nR\nV"
      # "R\nF\nU"
      # "R\nF\nU"
      # "R\nF\nU"
      # "H\nE\nA\nD\nE\nR"
      # "UTILITY"
      n78 = local read "Offset Pitch 2"() -> (w192:sgl)
      n79 = local read "LP_Z-North 2"() -> (w187:sgl)
      n80 = local read "Offset Yaw 2"() -> (w194:sgl)
      n81 = local read "LP_Y-Easth 2"() -> (w186:sgl)
      n82 = local read "Offset Roll 2"() -> (w193:sgl)
      n83 = local read "Longitude 2"() -> (w189:sgl)
      n84 = local read "Latitude  2"() -> (w190:sgl)
      n85 = local read "LP_X-Up 2"() -> (w185:sgl)
      n86 = local read "Azimuth 2"() -> (w191:sgl)
      n87 = local read "Height 2"() -> (w188:sgl)
      n88 = call "SGL-to-I16.vi"("Range"=w194) -> ("lo(x)"=w237:u8, "hi(x)"=w238:u8)  [unwired: 8 in, 1 out]
      n89 = call "SGL-to-I16.vi"("Range"=w193) -> ("lo(x)"=w235:u8, "hi(x)"=w236:u8)  [unwired: 8 in, 1 out]
      n90 = call "SGL-to-I16.vi"("Range"=w192) -> ("lo(x)"=w233:u8, "hi(x)"=w234:u8)  [unwired: 8 in, 1 out]
      n91 = call "SGL-to-IEEE754.vi"("Input_DBL"=w191) -> ("Output_U8"=w232:u8[])  [unwired: 10 in]
      n92 = call "SGL-to-IEEE754.vi"("Input_DBL"=w190) -> ("Output_U8"=w231:u8[])  [unwired: 10 in]
      n93 = call "SGL-to-IEEE754.vi"("Input_DBL"=w189) -> ("Output_U8"=w230:u8[])  [unwired: 10 in]
      n94 = call "SGL-to-IEEE754.vi"("Input_DBL"=w188) -> ("Output_U8"=w229:u8[])  [unwired: 10 in]
      n95 = call "SGL-to-IEEE754.vi"("Input_DBL"=w187) -> ("Output_U8"=w228:u8[])  [unwired: 10 in]
      n96 = call "SGL-to-IEEE754.vi"("Input_DBL"=w186) -> ("Output_U8"=w227:u8[])  [unwired: 10 in]
      n97 = call "SGL-to-IEEE754.vi"("Input_DBL"=w185) -> ("Output_U8"=w226:u8[])  [unwired: 10 in]
      n98 = Build Array(w179, FALSE ("element")) -> (w244:bool[], w178:bool, w177:bool, w176:bool)
      n99 = Build Array (concatenate)(u8 213, u8 90, u8 93, u8 85, w238, w237, w236, w235, w234, w233, w232, w231, w230, w229, w228, w227, w226) -> (w209:u8[])
      n100 = Boolean Array To Number(Boolean array=w244) -> (number=w243:u32)
      n101 = case shown="16" w243 {
        tunnel: [u8 0 u8 53 u8 189 u8 250 u8 238 u8 171] -> w180
        tunnel: [bool[] [] ("DV_Word") bool[] [TRUE, TRUE, TRUE, FALSE, FALSE, FALSE, FALSE, FALSE] ("DV_Word") bool[] [FALSE, FALSE, FALSE, FALSE, FALSE, FALSE, FALSE, TRUE] ("DV_Word") bool[] [FALSE, FALSE, FALSE, FALSE, FALSE, FALSE, TRUE, TRUE] ("DV_Word") bool[] [FALSE, FALSE, FALSE, FALSE, FALSE, FALSE, TRUE, TRUE] ("DV_Word") bool[] [FALSE, FALSE, FALSE, FALSE, FALSE, FALSE, TRUE, TRUE] ("DV_Word")] -> w181
        frame 0, Default {
        }
        frame 1 {
        }
        frame 2 {
        }
        frame 4 {
        }
        frame 8 {
        }
        frame 16 {
        }
      }
      n102 = Boolean Array To Number(Boolean array=w181) -> (number=w245:u32)
      n103 = Build Array(u8 0, u8 0, u8 3, u8 0) -> (w208:u8[])
      n104 = Build Array(u8 0, u8 0, u8 3, u8 0) -> (w207:u8[])
      n105 = Build Array(u8 0, u8 0, u8 3, u8 0) -> (w206:u8[])
      n106 = Build Array(u8 0, u8 3, u8 0, u8 0) -> (w205:u8[])
      n107 = To Unsigned Byte Integer(number=w245) -> (unsigned 8bit integer=w182:u8)
      n108 = Build Array (concatenate)(w209, w208, w207, w206, w205, w182, w180, w204, w203, w202) -> (w199:u8[])
      n109 = Byte Array To String(unsigned byte array=w199) -> (string=w201:string)
      n110 = call "crc16-ccitt (xFFFF).vi"("Message"=w201) -> ("CRC"=w200:u16)  [unwired: 9 in, 1 out]
      n111 = Split Number(x=w200) -> (hi(x)=w198:u8, lo(x)=w197:u8)
      n112 = Build Array (concatenate)(w199, w198, w197) -> (w196:u8[])
      n113 = Byte Array To String(unsigned byte array=w196) -> (string=w184:string)
    }
  }
  n114 = case shown="True" "Send" {
    tunnel: [_ w265] -> _
    tunnel: [_ w264] -> _
    tunnel: [_ w263] -> _
    tunnel: [_ w262] -> _
    tunnel: [_ "INIT"] -> _
    tunnel: [_ w260] -> _
    tunnel: [_ w259] -> _
    tunnel: [_ w258] -> _
    frame False {
    }
    frame True {
      w284 = u8 0  # ID3
      w285 = u8 0  # ID2
      w286 = u8 0  # ID1
      # "B#53"
      # "B#50"
      # "B#49"
      # "B#46"
      # "B#45"
      # "B#42"
      # "B#41"
      # "B#38"
      # "B#37"
      # "B#00"
      # "B_58"
      # "B_57"
      # "B_56"
      # "R\nE\nS\nE\nR\nV"
      # "R\nF\nU"
      # "R\nF\nU"
      # "R\nF\nU"
      # "H\nE\nA\nD\nE\nR"
      # "UTILITY"
      n115 = local read "Latitude  2"() -> (w272:sgl)
      n116 = local read "Offset Yaw 3"() -> (w276:sgl)
      n117 = local read "Offset Roll 3"() -> (w275:sgl)
      n118 = local read "Offset Pitch 3"() -> (w274:sgl)
      n119 = local read "Height 3"() -> (w270:sgl)
      n120 = local read "LP_Y-Easth 3"() -> (w268:sgl)
      n121 = local read "LP_X-Up 3"() -> (w267:sgl)
      n122 = local read "Azimuth 3"() -> (w273:sgl)
      n123 = local read "Longitude 3"() -> (w271:sgl)
      n124 = local read "LP_Z-North 3"() -> (w269:sgl)
      n125 = call "SGL-to-I16.vi"("Range"=w276) -> ("lo(x)"=w319:u8, "hi(x)"=w320:u8)  [unwired: 8 in, 1 out]
      n126 = call "SGL-to-I16.vi"("Range"=w275) -> ("lo(x)"=w317:u8, "hi(x)"=w318:u8)  [unwired: 8 in, 1 out]
      n127 = call "SGL-to-I16.vi"("Range"=w274) -> ("lo(x)"=w315:u8, "hi(x)"=w316:u8)  [unwired: 8 in, 1 out]
      n128 = call "SGL-to-IEEE754.vi"("Input_DBL"=w273) -> ("Output_U8"=w314:u8[])  [unwired: 10 in]
      n129 = call "SGL-to-IEEE754.vi"("Input_DBL"=w272) -> ("Output_U8"=w313:u8[])  [unwired: 10 in]
      n130 = call "SGL-to-IEEE754.vi"("Input_DBL"=w271) -> ("Output_U8"=w312:u8[])  [unwired: 10 in]
      n131 = call "SGL-to-IEEE754.vi"("Input_DBL"=w270) -> ("Output_U8"=w311:u8[])  [unwired: 10 in]
      n132 = call "SGL-to-IEEE754.vi"("Input_DBL"=w269) -> ("Output_U8"=w310:u8[])  [unwired: 10 in]
      n133 = call "SGL-to-IEEE754.vi"("Input_DBL"=w268) -> ("Output_U8"=w309:u8[])  [unwired: 10 in]
      n134 = call "SGL-to-IEEE754.vi"("Input_DBL"=w267) -> ("Output_U8"=w308:u8[])  [unwired: 10 in]
      n135 = Build Array(FALSE ("element"), FALSE ("element")) -> (w326:bool[], w265:bool, w264:bool, w263:bool)
      n136 = Boolean Array To Number(Boolean array=w326) -> (number=w325:u32)
      n137 = Build Array (concatenate)(u8 213, u8 90, u8 93, u8 85, w320, w319, w318, w317, w316, w315, w314, w313, w312, w311, w310, w309, w308) -> (w291:u8[])
      n138 = case shown="2" w325 {
        tunnel: [u8 0 u8 53 u8 189 u8 250 u8 238 u8 171] -> w258
        tunnel: [bool[] [] ("DV_Word") bool[] [TRUE, TRUE, TRUE, FALSE, FALSE, FALSE, FALSE, FALSE] ("DV_Word") bool[] [FALSE, FALSE, FALSE, FALSE, FALSE, FALSE, FALSE, TRUE] ("DV_Word") bool[] [FALSE, FALSE, FALSE, FALSE, FALSE, FALSE, TRUE, TRUE] ("DV_Word") bool[] [FALSE, FALSE, FALSE, FALSE, FALSE, FALSE, TRUE, TRUE] ("DV_Word") bool[] [FALSE, FALSE, FALSE, FALSE, FALSE, FALSE, TRUE, TRUE] ("DV_Word")] -> w259
        frame 0, Default {
        }
        frame 1 {
        }
        frame 2 {
        }
        frame 4 {
        }
        frame 8 {
        }
        frame 16 {
        }
      }
      n139 = Boolean Array To Number(Boolean array=w259) -> (number=w327:u32)
      n140 = To Unsigned Byte Integer(number=w327) -> (unsigned 8bit integer=w260:u8)
      n141 = Build Array(u8 15, u8 30, u8 45, u8 60) -> (w290:u8[])
      n142 = Build Array(u8 75, u8 90, u8 105, u8 120) -> (w289:u8[])
      n143 = Build Array(u8 135, u8 150, u8 165, u8 180) -> (w288:u8[])
      n144 = Build Array(u8 3, u8 3, u8 3, u8 3) -> (w287:u8[])
      n145 = Build Array (concatenate)(w291, w290, w289, w288, w287, w260, w258, w286, w285, w284) -> (w281:u8[])
      n146 = Byte Array To String(unsigned byte array=w281) -> (string=w283:string)
      n147 = call "crc16-ccitt (xFFFF).vi"("Message"=w283) -> ("CRC"=w282:u16)  [unwired: 9 in, 1 out]
      n148 = Split Number(x=w282) -> (hi(x)=w280:u8, lo(x)=w279:u8)
      n149 = Build Array (concatenate)(w281, w280, w279) -> (w278:u8[])
      n150 = Byte Array To String(unsigned byte array=w278) -> (string=w262:string)
    }
  }
  n151 = VISA Close(VISA resource name=w8, error in (no error)=w7) -> ()  [unwired: 1 out]
